vi "Do.vi"(8 "error in (no error)":errorcluster, 10 "Actor in":refnum<class "Actor.lvclass">, 11 "Actor Launched Msg":refnum<class "Actor Launched Msg.lvclass">) -> (0 "error out":errorcluster, 2 "Actor out":refnum<class "Actor.lvclass">)   [LabVIEW 2018, in "Monitored Actor.lvlib" / "Actor Launched Msg.lvclass"]
doc: "This VI delivers the message to the actor by calling the appropriate method(s) on the actor."
uses:
  Actor Launched Msg.lvclass
  <vilib>/ActorFramework/Actor/Actor.lvclass
  Actor/Actor Monitor.lvclass
  C:/Program Files (x86)/National Instruments/LabVIEW 2018/vi.lib/ActorFramework/Actor/Actor.lvclass
  Actor Launched Msg.lvclass/Actor Launched Msg.ctl
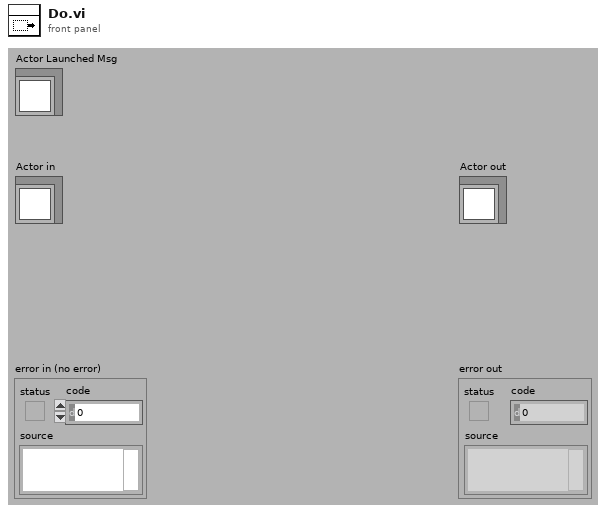
[diagram p1: front panel]
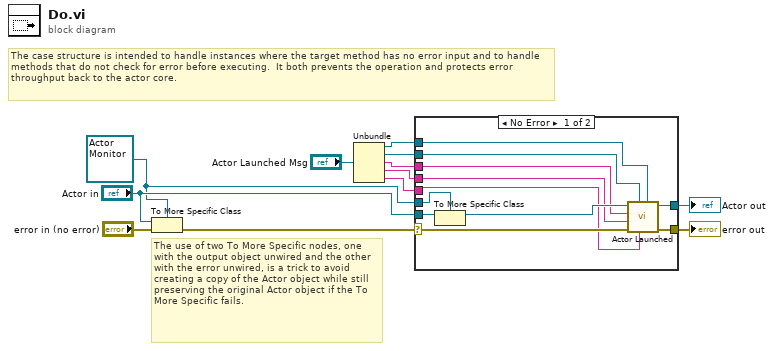
[diagram p0: block diagram]
diagram:
  w6 = refnum<class "Actor Monitor.lvclass"> refnum ("Actor in")
  # "The use of two To More Specific nodes, one with the output object unwired and the other with the error unwired, is a trick to avoid creating a copy of the Actor object while still preserving the original Actor object if the To More Specific fails."
  # "The case structure is intended to handle instances where the target method has no error input and to handle methods that do not check for error before executing.  It both prevents the operation and protects error throughput back to the actor core."
  n1 = To More Specific Class(target class=w6, reference="Actor in", error in="error in (no error)") -> (error out=w10:errorcluster)  [unwired: 1 out]
  n2 = Unbundle("Actor Launched Msg") -> (w5:refnum<class "Message Enqueuer.lvclass">, w4:refnum<class "Message Enqueuer.lvclass">, w3:string, w2:string, w1:string)
  n3 = case shown="No Error" w10 {
    selector: w10 -> [w21 w25]
    tunnel: [w23 w25] -> w9
    tunnel: [w22 w24] -> w8
    tunnel: "Actor in" -> [w20 w24]
    tunnel: w6 -> [w19 _]
    tunnel: w5 -> [w17 _]
    tunnel: w4 -> [w16 _]
    tunnel: w3 -> [w15 _]
    tunnel: w2 -> [w14 _]
    tunnel: w1 -> [w13 _]
    frame No Error {
      n4 = To More Specific Class(target class=w19, reference=w20) -> (specific class reference=w18:refnum<class "Actor Monitor.lvclass">)  [unwired: 1 in, 1 out]
      n5 = call "Actor Launched.vi"("Actor's Caller"=w17, "Actor Core Name"=w13, "Actor's Queue"=w16, "error in (no error)"=w21, "Actor ID"=w14, "Class Name"=w15, "Actor Monitor in"=w18) -> ("error out"=w23:errorcluster, "Actor Monitor out"=w22:refnum<class "Actor Monitor.lvclass">)  [unwired: 3 in]
    }
    frame Error {
      # "If type check fails, pass the original object out again."
    }
  }
  "error out" <- w9
  "Actor out" <- w8
